vi "RoundI64.vi"(5 "Decimal places":i8, 6 "Number":i64) -> (2 "Rounded number":i64)   [LabVIEW 2017, in "GPNumeric.lvlib"]
doc: "Rounds <B>Number</B> to a number of <B>Decimal places</B>.\n\nSet <B>Decimal places</B> to a negative number to round to nearest 10, nearest 100 and so on. E.g. to round 782 to the nearest hundred, you set <B>Decimal places</B> to -2 and the <B>Rounded number</B> will be 800.\n\nThis VI is inlined.\n\n<B>Note</B> This VI uses the default IEEE 754 round-half-to-even rounding mode.\n\nSteen Schmidt\nGPower\n14/5 2014"
uses:
  GPNumeric.lvlib
  Overflow/GPOverflow.lvlib
  Overflow/Library/Mult/MultI64.vi
panel:
  # "Copyright © 2014\nGPower\nSee enclosed license file for terms and conditions"
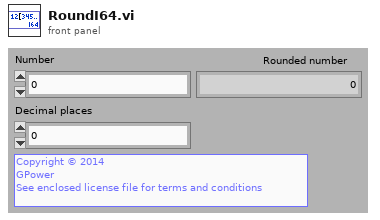
[diagram p1: front panel]
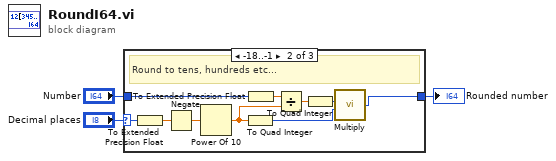
[diagram p0: block diagram]
diagram:
  n1 = case shown="-18..-1" "Decimal places" {
    selector: "Decimal places" -> [_ w8 _]
    tunnel: [_ w5 w14] -> w3
    tunnel: "Number" -> [_ w6 w14]
    frame ..-19 {
      # "Round above max value; Return zero."
    }
    frame -18..-1 {
      # "Round to tens, hundreds etc..."
      n2 = To Extended Precision Float(1:w8) -> (0:w7:ext)
      n3 = Negate(x=w7) -> (-x=w13:ext)
      n4 = Power Of 10(x=w13) -> (10^x=w4:ext)
      n5 = To Quad Integer(1:w4) -> (0:w11:i64)
      n6 = To Extended Precision Float(1:w6) -> (0:w9:ext)
      n7 = Divide(x=w9, y=w4) -> (x/y=w12:ext)
      n8 = To Quad Integer(1:w12) -> (0:w10:i64)
      n9 = call-poly "Multiply.vi"("y"=w11, "x"=w10) -> ("x*y"=w5:i64)  [unwired: 3 in, 1 out]
    }
    frame 0.. {
      # "Round to n decimal places; return integer unchanged."
    }
  }
  "Rounded number" <- w3
